vi "DriveStateMachine.vi"   [LabVIEW 2018]
uses:
  DriveLoopEnum.ctl
  <vilib>/Rock Robotics/WPI/Utilities/WPI_GetSetVariantRefNum.vi
types:
  T1 = typedef "DriveLoopEnum.ctl" = enum16{"Manual", "Motion Magic"}
  T2 = typedef "WPI_JoystickDevRef.ctl" = cluster{"Device":T3}
  T3 = typedef "WPI_JoystickDeviceEnum.ctl" = enum16{"USB 0", "USB 1", "USB 2", "USB 3", "USB 4", "USB 5"}
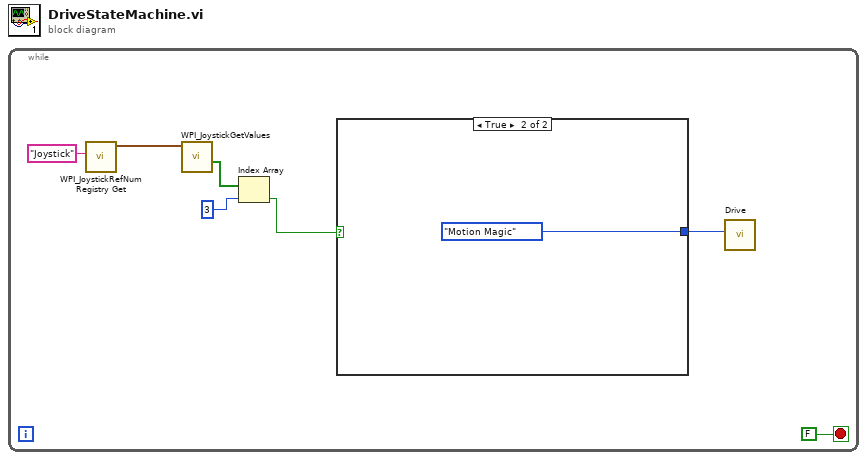
[diagram p0: block diagram]
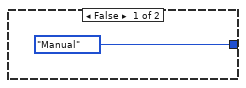
[diagram p2: hidden frame]
diagram:
  n1 = while {
    stop <- FALSE stop-if-true
    n2 = call <vilib>:"WPI_JoystickRefNum Registry Get.vi"("refnum name"="Joystick") -> ("JoystickDevRef"=w6:T2)  [unwired: 9 in, 1 out]
    n3 = call <vilib>:"WPI_JoystickGetValues.vi"("JoystickDevRef"=w6) -> ("Buttons"=w5:bool[])  [unwired: 6 in, 4 out]
    n4 = Index Array(array=w5, index=3) -> (element=w4:bool)
    n5 = case shown="True" w4 {
      tunnel: [DriveLoopEnum."Manual" ("Drive Loop State") DriveLoopEnum."Motion Magic" ("Drive Loop State")] -> w3
      frame False {
      }
      frame True {
      }
    }
    n6 = call "Drive.vi"("Drive Loop State"=w3) -> ()  [unwired: 11 in]
  }
